vi "AutoConfigYScales.vi"(9 "Y标尺总数":i32, 10 "已选信号数组":refnum<vi>, 11 "XYGraph输入":refnum<vi>) -> ()   [LabVIEW 2015]
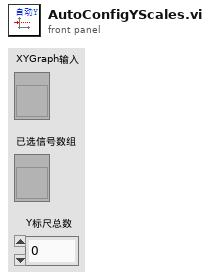
[diagram p1: front panel]
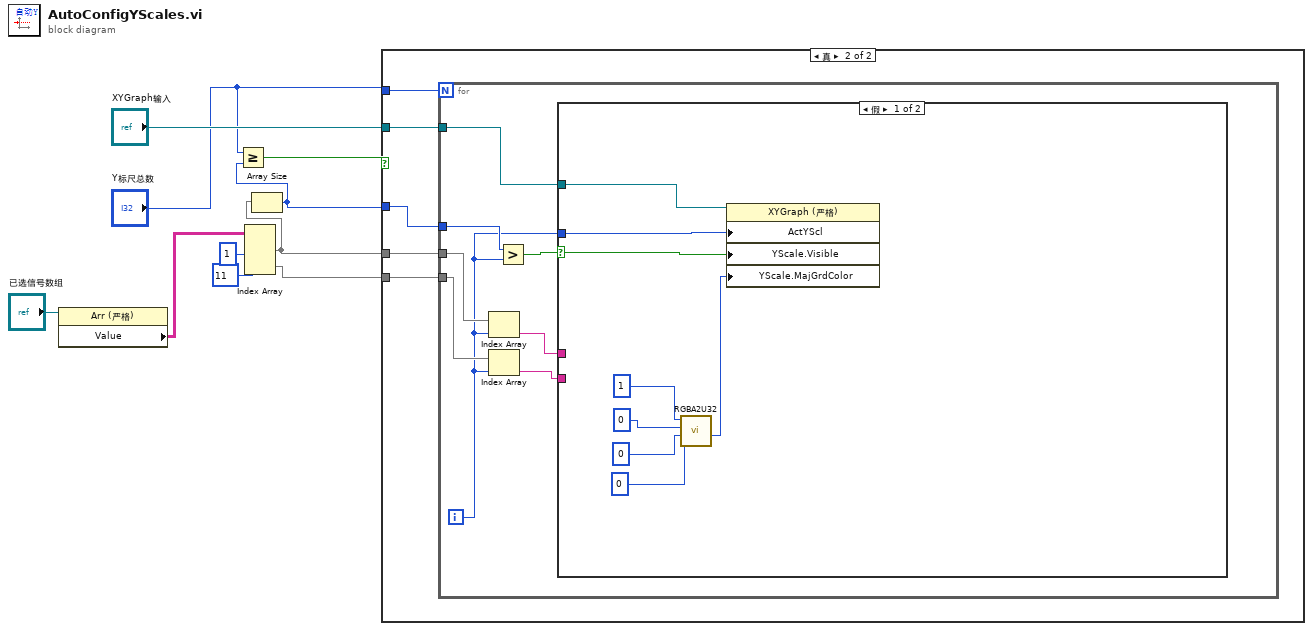
[diagram p0: block diagram]
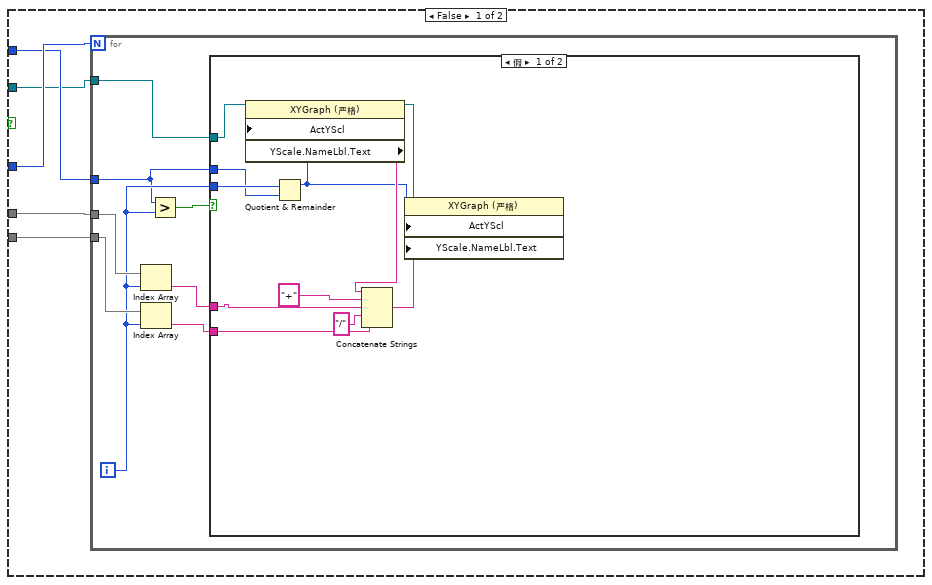
[diagram p2: hidden frame]
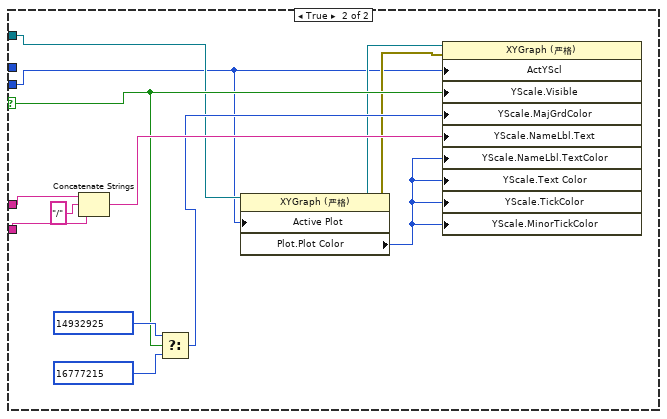
[diagram p3: hidden frame]
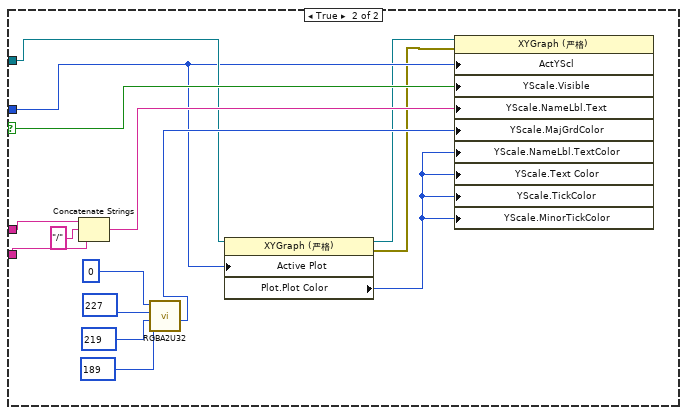
[diagram p4: hidden frame]
diagram:
  n1 = property class="Arr (严格)"(reference="已选信号数组") -> ("Value"=w2:string[][])  [unwired: 1 in, 2 out]
  n2 = Index Array(array=w2, index (col) #1=1 ("禁用的索引 (列)"), index (col) #2=11 ("索引 (列)")) -> (element #1=w7:string[], element #2=w8:string[])  [unwired: 2 in]
  n3 = Array Size(array=w7) -> (size(s)=w9:i32)
  n4 = Greater Or Equal?(x="Y标尺总数", y=w9) -> (x >= y?=w4:bool)
  n5 = case shown="真" w4 {
    tunnel: "Y标尺总数" -> [w12 w52]
    tunnel: w7 -> [w14 w51]
    tunnel: w8 -> [w15 w50]
    tunnel: w9 -> [w13 w49]
    tunnel: "XYGraph输入" -> [w11 w48]
    frame False {
      n6 = for {
        N: w13 -> [_]
        tunnel: w14 -> [w20]
        tunnel: w15 -> [w19]
        tunnel: w12 -> [w16]
        tunnel: w11 -> [w18]
        i -> [w17]
        n7 = Index Array(array=w20, index=w17) -> (element=w22:string)
        n8 = Index Array(array=w19, index=w17) -> (element=w21:string)
        n9 = Greater?(x=w16, y=w17) -> (0:w23:bool)
        n10 = case shown="假" w23 {
          selector: w23 -> [_ w41]
          tunnel: w18 -> [w34 w39]
          tunnel: w17 -> [w33 w36]
          tunnel: w22 -> [w30 w44]
          tunnel: w21 -> [w29 w47]
          tunnel: w16 -> [w32 _]
          frame False {
            n11 = Quotient & Remainder(x=w33, y=w32) -> (x-y*floor(x/y)=w25:i32)  [unwired: 1 out]
            n12 = property class="XYGraph (严格)"(reference=w34, "ActYScl"=w25) -> (reference out=w26:refnum<vi>, "YScale.NameLbl.Text"=w28:string)  [unwired: 1 in, 1 out]
            n13 = Concatenate Strings(w28, "+" ("字符串"), w30, "/" ("字符串"), w29) -> (w24:string)
            n14 = property class="XYGraph (严格)"(reference=w26, "ActYScl"=w25, "YScale.NameLbl.Text"=w24) -> ()  [unwired: 1 in, 2 out]
          }
          frame True {
            n15 = Concatenate Strings(w44, "/" ("字符串"), w47) -> (w46:string)
            n16 = Select(t=u32 14932925 ("Y标尺.网格颜色:主网格颜色"), s=w41, f=u32 16777215 ("Y标尺.网格颜色:主网格颜色")) -> (s? t:f=w40:u32)
            n17 = property class="XYGraph (严格)"(reference=w39, "Active Plot"=w36) -> (reference out=w38:refnum<vi>, error out=w37:errorcluster, "Plot.Plot Color"=w35:u32)  [unwired: 1 in]
            n18 = property class="XYGraph (严格)"(reference=w38, error in=w37, "ActYScl"=w36, "YScale.Visible"=w41, "YScale.MajGrdColor"=w40, "YScale.NameLbl.Text"=w46, "YScale.NameLbl.TextColor"=w35, "YScale.Text Color"=w35, "YScale.TickColor"=w35, "YScale.MinorTickColor"=w35) -> ()  [unwired: 2 out]
          }
        }
      }
    }
    frame True {
      n19 = for {
        N: w52 -> [_]
        tunnel: w51 -> [w57]
        tunnel: w50 -> [w56]
        tunnel: w49 -> [w55]
        tunnel: w48 -> [w54]
        i -> [w53]
        n20 = Index Array(array=w57, index=w53) -> (element=w59:string)
        n21 = Index Array(array=w56, index=w53) -> (element=w58:string)
        n22 = Greater?(x=w55, y=w53) -> (0:w60:bool)
        n23 = case shown="假" w60 {
          selector: w60 -> [w66 w79]
          tunnel: w54 -> [w68 w73]
          tunnel: w53 -> [w67 w72]
          tunnel: w59 -> [_ w80]
          tunnel: w58 -> [_ w83]
          frame False {
            n24 = call "RGBA2U32.vi"("B(0to255)"=u8 0, "G(0to255)"=u8 0, "R(0to255)"=u8 0, "Transparency (0or1)"=u8 1) -> ("ColorU32"=w61:u32)  [unwired: 6 in]
            n25 = property class="XYGraph (严格)"(reference=w68, "ActYScl"=w67, "YScale.Visible"=w66, "YScale.MajGrdColor"=w61) -> ()  [unwired: 1 in, 2 out]
          }
          frame True {
            n26 = Concatenate Strings(w80, "/" ("字符串"), w83) -> (w82:string)
            n27 = call "RGBA2U32.vi"("B(0to255)"=u8 189, "G(0to255)"=u8 219, "R(0to255)"=u8 227, "Transparency (0or1)"=u8 0) -> ("ColorU32"=w74:u32)  [unwired: 6 in]
            n28 = property class="XYGraph (严格)"(reference=w73, "Active Plot"=w72) -> (reference out=w71:refnum<vi>, error out=w70:errorcluster, "Plot.Plot Color"=w69:u32)  [unwired: 1 in]
            n29 = property class="XYGraph (严格)"(reference=w71, error in=w70, "ActYScl"=w72, "YScale.Visible"=w79, "YScale.NameLbl.Text"=w82, "YScale.MajGrdColor"=w74, "YScale.NameLbl.TextColor"=w69, "YScale.Text Color"=w69, "YScale.TickColor"=w69, "YScale.MinorTickColor"=w69) -> ()  [unwired: 2 out]
          }
        }
      }
    }
  }
